vi "fit elliptical orbit to many magnetometer readings multi-stage.vi"(0 "initial parameters 1":T1, 1 "fixed parameters":T1={"a"=nan, "b"=nan, "theta_axis"=nan, "dPhi"=nan, "BrV"=nan, "bob tilt"=nan, "phi0"=nan, "phi_dot"=nan, "x0"=nan, "y0"=nan, "z0"=nan}, 5 "initial parameters 2":T1, 7 "magnetometer readings":T3[](array[typedef]), 9 "omega":dbl, 11 "t0":dbl) -> (4 "fit parameters":T1, 6 "error":bool, 8 "residue":dbl, 12 "set 1 selected":bool, 15 "fit graph":T2(array[cluster]))   [LabVIEW 2017]
uses:
  typedefs/orbit parameters full.ctl
  typedefs/magnetomter reading set.ctl
panel:
  out "number of function calls 2":i32
  out "number of function calls":i32
  out "error 2":bool
  out "residue 2":dbl
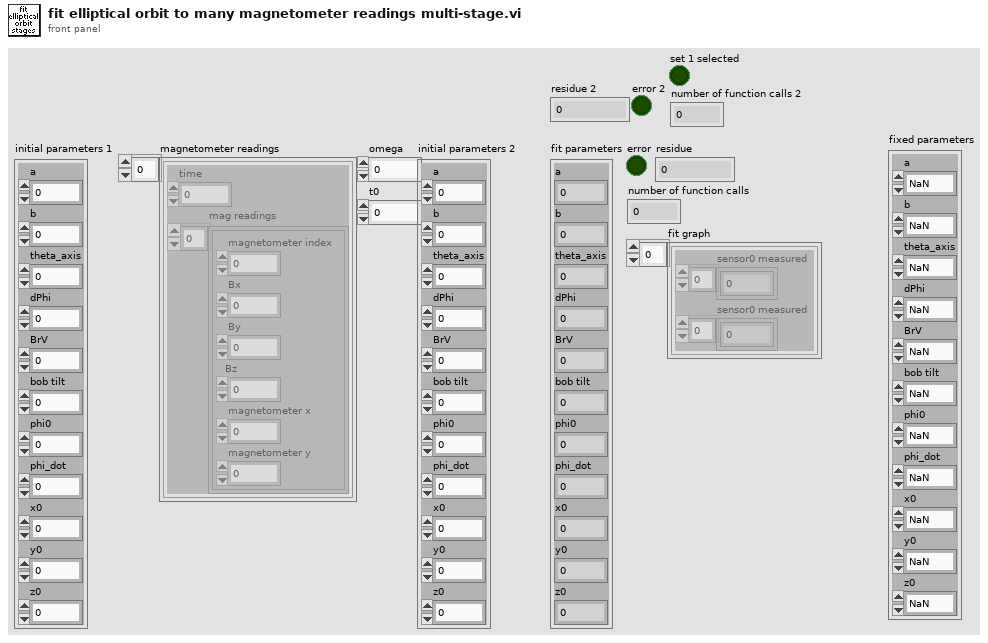
[diagram p1: front panel]
types:
  T1 = typedef "orbit parameters full.ctl" = cluster{"a":dbl, "b":dbl, "theta_axis":dbl, "dPhi":dbl, "BrV":dbl, "bob tilt":dbl, "phi0":dbl, "phi_dot":dbl, "x0":dbl, "y0":dbl, "z0":dbl}
  T2 = cluster{"sensor0 measured":dbl[], "sensor0 measured":dbl[]}[]
  T3 = typedef "magnetomter reading set.ctl" = cluster{"time":fxp<+,48,48>, "mag readings":cluster{"magnetometer index":dbl, "Bx":dbl, "By":dbl, "Bz":dbl, "magnetometer x":dbl, "magnetometer y":dbl}[]}
  T4 = cluster{"[0]":dbl, "[1]":dbl, "[2]":dbl, "[3]":dbl, "[4]":dbl, "[5]":dbl, "[6]":dbl, "[7]":dbl, "[8]":dbl, "[9]":dbl, "[10]":dbl}
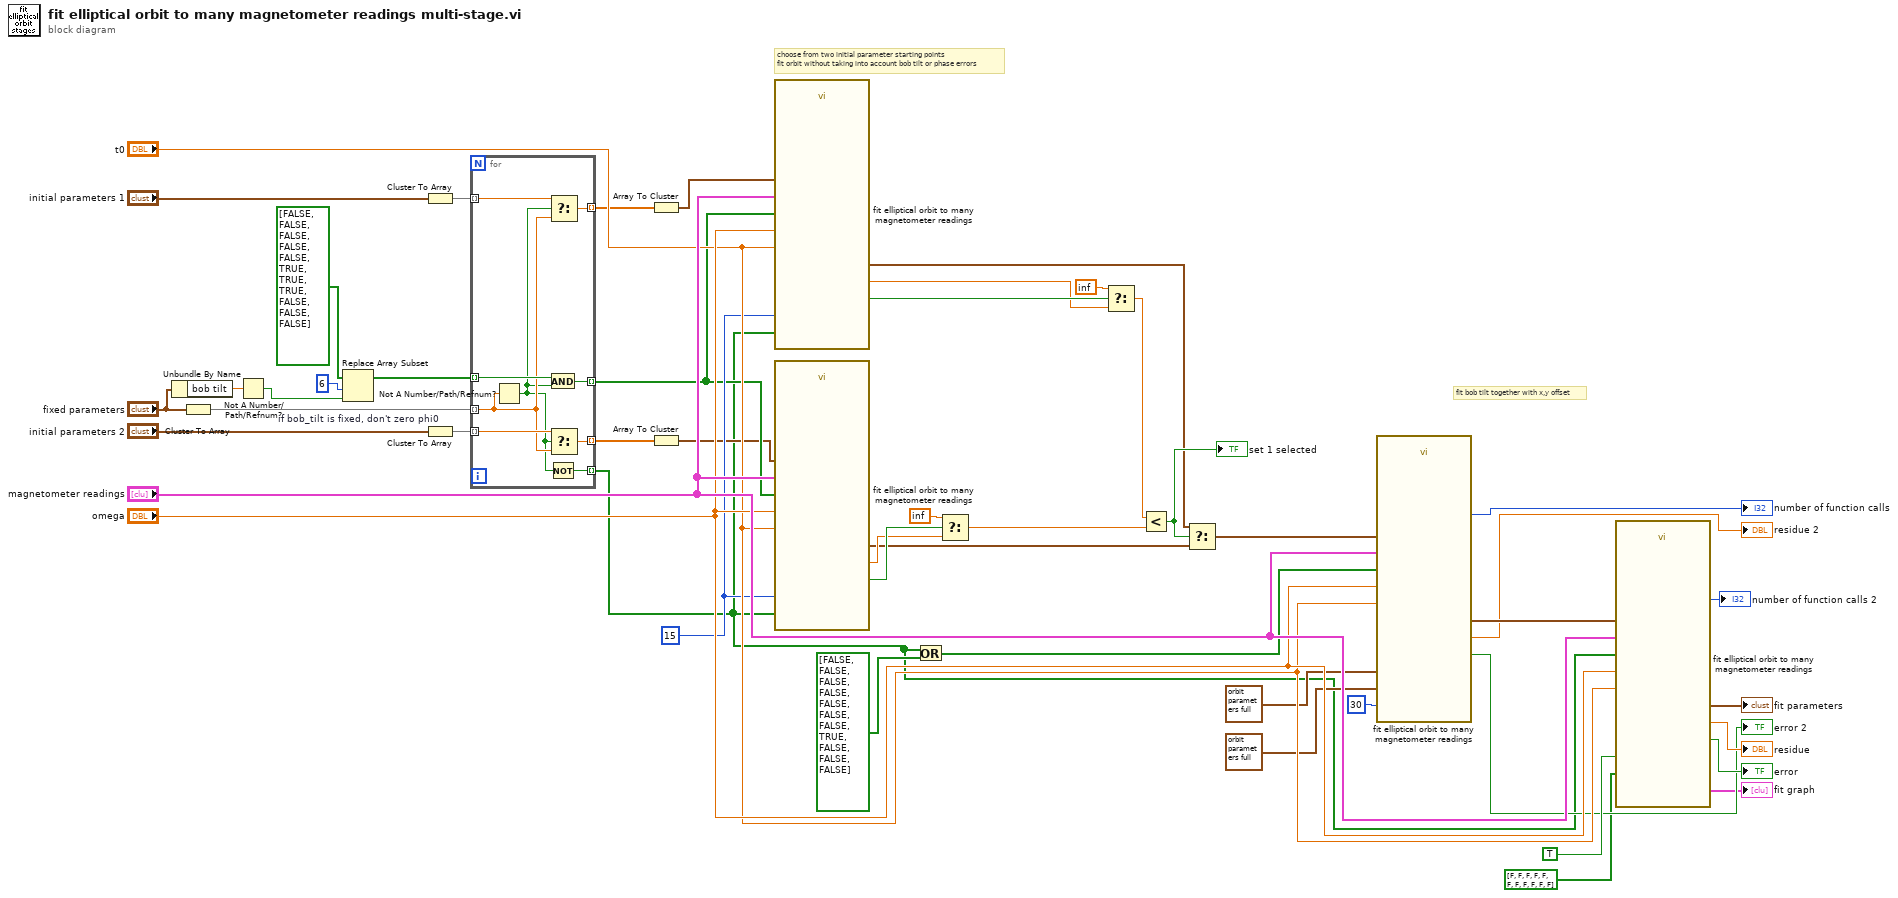
[diagram p0: block diagram]
diagram:
  w21 = 15 ("max readings to fit")
  # "fit bob tilt together with x,y offset"
  # "choose from two initial parameter starting points\nfit orbit without taking into account bob tilt or phase errors"
  n1 = Unbundle By Name("fixed parameters") -> ("bob tilt"=w6:dbl)
  n2 = Cluster To Array(cluster="fixed parameters") -> (array=w19:dbl[])
  n3 = Not A Number/Path/Refnum?(number/path/refnum=w6) -> (NaN/Path/Refnum?=w3:bool)
  n4 = Replace Array Subset "if bob_tilt is fixed, don't zero phi0"(array=bool[] [FALSE, FALSE, FALSE, FALSE, FALSE, TRUE, TRUE, TRUE, FALSE, FALSE, FALSE] ("zero parameter"), new element=w3, index=6) -> (w4:bool[])
  n5 = Cluster To Array(cluster="initial parameters 1") -> (array=w18:dbl[])
  n6 = Cluster To Array(cluster="initial parameters 2") -> (array=w16:dbl[])
  n7 = for {
    tunnel: w19 -> [w53] mode=indexing
    tunnel: w18 -> [w56] mode=indexing
    tunnel: w16 -> [w54] mode=indexing
    tunnel: w4 -> [w58] mode=indexing
    tunnel: [w57] -> w15 mode=indexing
    tunnel: [w55] -> w12 mode=indexing
    tunnel: [w52] -> w14 mode=indexing
    tunnel: [w50] -> w8 mode=indexing
    n8 = Not A Number/Path/Refnum?(number/path/refnum=w53) -> (NaN/Path/Refnum?=w51:bool)
    n9 = And(x=w58, y=w51) -> (x .and. y?=w57:bool)
    n10 = Not(x=w51) -> (.not. x?=w50:bool)
    n11 = Select(t=w56, s=w51, f=w53) -> (s? t:f=w55:dbl)
    n12 = Select(t=w54, s=w51, f=w53) -> (s? t:f=w52:dbl)
  }
  n13 = Array To Cluster(array=w12) -> (cluster=w10:T4)
  n14 = Array To Cluster(array=w14) -> (cluster=w13:T4)
  n15 = call "fit elliptical orbit to many magnetometer readings.vi"("initial parameters"=w10, "magnetometer readings"="magnetometer readings", "fix parameter?"=w8, "omega"="omega", "t0"="t0", "max readings to fit"=w21, "zero parameter"=w15) -> ("error"=w49:bool, "fit parameters"=w40:T1, "residue"=w48:dbl)  [unwired: 3 in, 7 out]
  n16 = call "fit elliptical orbit to many magnetometer readings.vi"("initial parameters"=w13, "magnetometer readings"="magnetometer readings", "fix parameter?"=w8, "omega"="omega", "t0"="t0", "max readings to fit"=w21, "zero parameter"=w15) -> ("error"=w46:bool, "fit parameters"=w39:T1, "residue"=w45:dbl)  [unwired: 3 in, 7 out]
  n17 = Or(x=w8, y=bool[] [FALSE, FALSE, FALSE, FALSE, FALSE, FALSE, FALSE, TRUE, FALSE, FALSE, FALSE] ("fix parameter?")) -> (x .or. y?=w9:bool[])
  n18 = Select(t=inf, s=w46, f=w45) -> (s? t:f=w42:dbl)
  n19 = Select(t=inf, s=w49, f=w48) -> (s? t:f=w43:dbl)
  n20 = Less?(x=w43, y=w42) -> (x < y?=w41:bool)
  "set 1 selected" <- w41
  n21 = Select(t=w40, s=w41, f=w39) -> (s? t:f=w38:T1)
  n22 = call "fit elliptical orbit to many magnetometer readings.vi"("initial parameters"=w38, "magnetometer readings"="magnetometer readings", "fix parameter?"=w9, "omega"="omega", "t0"="t0", "maximums"=T1 {"a"=300.0, "b"=300.0, "theta_axis"=7.0, "dPhi"=0.1, "BrV"=10000.0, "bob tilt"=0.3, "phi0"=3.0, "phi_dot"=7.0, "x0"=4.0, "y0"=4.0, "z0"=200.0}, "minimums"=T1 {"a"=0.0, "b"=-300.0, "theta_axis"=-7.0, "dPhi"=-0.1, "BrV"=-10000.0, "bob tilt"=-0.3, "phi0"=3.0, "phi_dot"=-7.0, "x0"=-4.0, "y0"=-4.0, "z0"=-200.0}, "max readings to fit"=30) -> ("number of function calls"=→"number of function calls":i32, "error"=→"error 2":bool, "fit parameters"=w37:T1, "residue"=→"residue 2":dbl)  [unwired: 2 in, 6 out]
  n23 = call "fit elliptical orbit to many magnetometer readings.vi"("initial parameters"=w37, "magnetometer readings"="magnetometer readings", "extra precision"=TRUE, "fix parameter?"=w8, "omega"="omega", "t0"="t0", "zero parameter"=bool[] [FALSE, FALSE, FALSE, FALSE, FALSE, FALSE, FALSE, FALSE, FALSE, FALSE, FALSE]) -> ("number of function calls"=→"number of function calls 2":i32, "error"=→"error":bool, "fit parameters"=→"fit parameters":T1, "fit graph"=→"fit graph":T2, "residue"=→"residue":dbl)  [unwired: 3 in, 5 out]
